vi "Write Headers.vi"(8 "error in":errorcluster, 11 "CSV in":refnum<class "CSV.lvclass">) -> (0 "error out":errorcluster, 3 "CSV out":refnum<class "CSV.lvclass">)   [LabVIEW 2020, in "Manejador archivo.lvlib" / "CSV.lvclass"]
uses:
  CSV.lvclass
  C:/GitClones/DQMH-LabVIEW-GYM/10 Mayo/04 DQMH USER/Libraries/Manejador archivo/Class Definitions/File/File.lvclass
  CSV.lvclass/CSV.ctl
  File/File.lvclass/File.ctl
  File/Read Delimiter.vi
  Read file Ref.vi
  File/Read Column Headers.vi
  File/Read Save Timestamp.vi
  Write Headers_.vi
  Read Headers_.vi
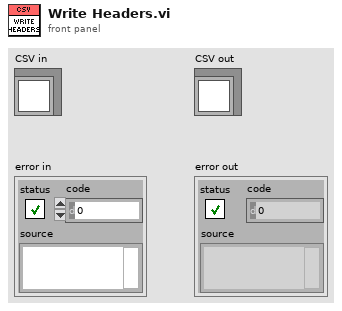
[diagram p1: front panel]
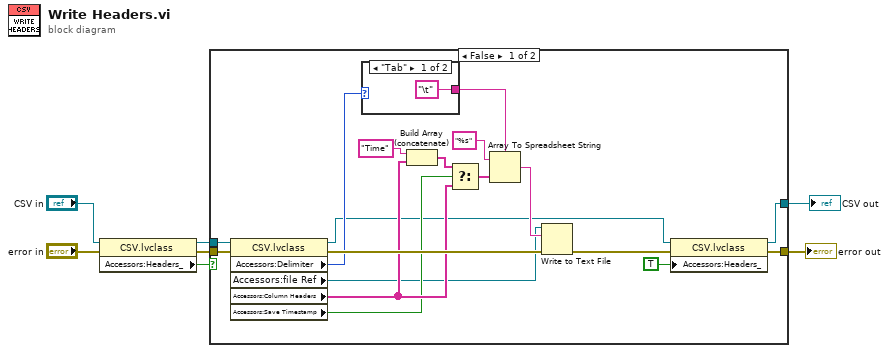
[diagram p0: block diagram]
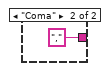
[diagram p2: hidden frame]
diagram:
  n1 = property class="CSV.lvclass"(reference="CSV in", error in="error in") -> (reference out=w2:refnum<class "CSV.lvclass">, error out=w5:errorcluster, "Accessors:Headers_"=w1:bool)
  n2 = case shown="False" w1 {
    tunnel: [w23 w29] -> w6
    tunnel: [w10 w28] -> w4
    tunnel: w5 -> [w22 w29]
    tunnel: w2 -> [w8 w28]
    frame False {
      n3 = property class="CSV.lvclass"(reference=w8, error in=w22) -> (reference out=w11:refnum<class "CSV.lvclass">, error out=w25:errorcluster, "Accessors:Delimiter"=w13:enum16{"Tab", "Coma"}, "Accessors:file Ref"=w14:refnum<file>, "Accessors:Column Headers"=w16:string[], "Accessors:Save Timestamp"=w15:bool)
      n4 = case shown="\"Tab\"" w13 {
        tunnel: ["\t" ","] -> w12
        frame "Tab" {
        }
        frame "Coma" {
        }
      }
      n5 = Build Array (concatenate)("Time", w16) -> (w18:string[])
      n6 = Select(t=w18, s=w15, f=w16) -> (s? t:f=w20:string[])
      n7 = Array To Spreadsheet String(delimiter (Tab)=w12, array=w20, 3:"%s" ("format string")) -> (spreadsheet string=w21:string)
      n8 = Write to Text File(file (use dialog)=w14, text=w21, error in=w25) -> (error out=w24:errorcluster)  [unwired: 1 in, 2 out]
      n9 = property class="CSV.lvclass"(reference=w11, error in=w24, "Accessors:Headers_"=TRUE ("Headers_")) -> (reference out=w10:refnum<class "CSV.lvclass">, error out=w23:errorcluster)
    }
    frame True {
    }
  }
  "error out" <- w6
  "CSV out" <- w4
